vi "MENG4730 Flow Control By Valve Experiment.vi"() -> ()   [LabVIEW 2021]
uses:
  <vilib>/addons/control/pid/pid.llb/PID (DBL).vi
  <vilib>/Modbus/slave/Modbus Slave.lvclass
  <vilib>/addons/control/pid/NI_PID_pid.lvlib
panel:
  in  "FV1":bool
  out "x+1":dbl
  out "FV2":sgl
  out "F1 Values Array":dbl[](array[numeric])
  out "output":sgl
  in  "Flow Setpoint":dbl format="%.2f"
  out "Waveform Graph":sgl[](graph)
  in  "PID gains":T1={"proportional gain (Kc)"=1.0, "integral time (Ti, min)"=0.01, "derivative time (Td, min)"=0.0} {"derivative time (Td, min)" format="%.3f"; "integral time (Ti, min)" format="%.3f"; "proportional gain (Kc)" format="%.3f"}
  out "F1":sgl
  out "F1":sgl(knob) scale=0.0..100.0
  in  "stop":bool
  in  "M1":sgl(slide) scale=0.0..100.0
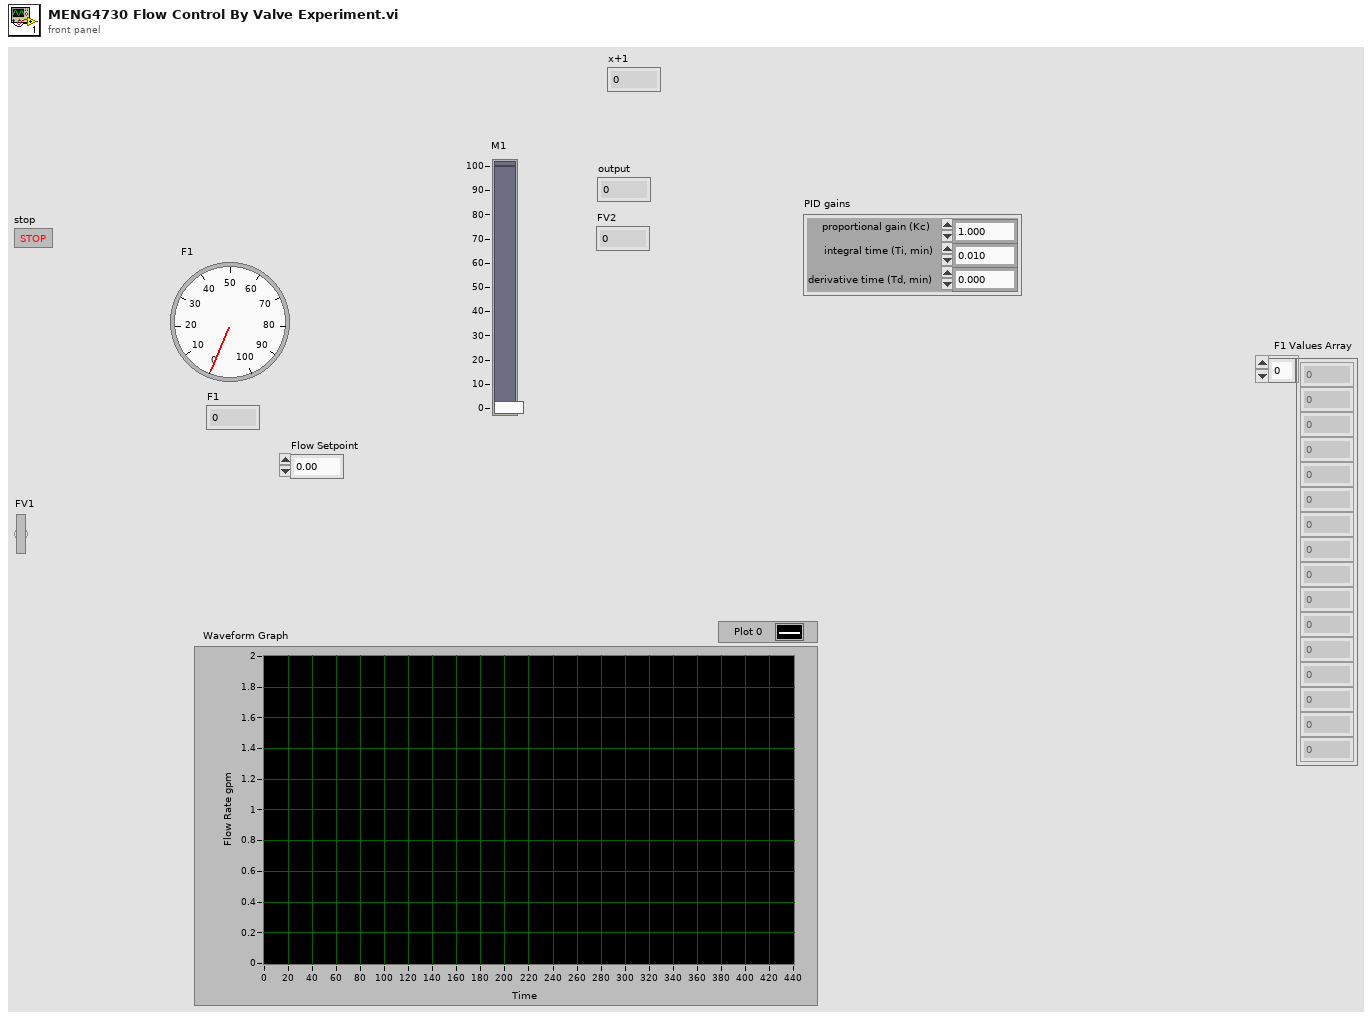
[diagram p1: front panel]
types:
  T1 = cluster{"proportional gain (Kc)":dbl, "integral time (Ti, min)":dbl, "derivative time (Td, min)":dbl}
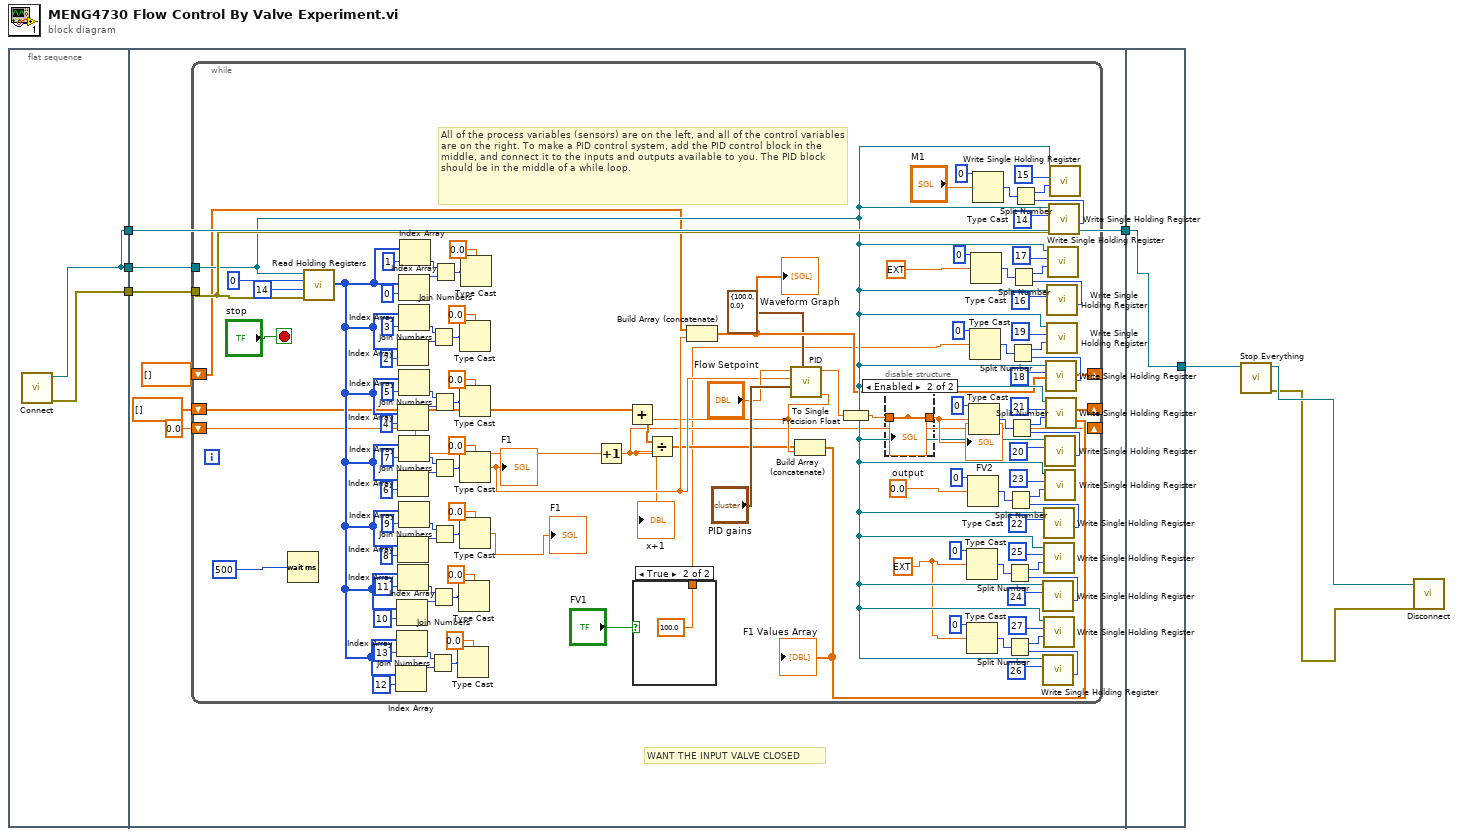
[diagram p0: block diagram]
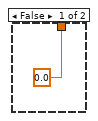
[diagram p2: hidden frame]
diagram:
  n1 = flat-sequence {
    tunnel: [w9] -> w7
    tunnel: [w8] -> w6
    tunnel: [w9] -> w5
    tunnel: w7 -> [w15]
    tunnel: w6 -> [w14]
    tunnel: [w13] -> w4
    tunnel: w5 -> [w13]
    tunnel: w4 -> [w133]
    tunnel: [w133] -> w3
    frame #0 {
      n2 = call "Connect.vi"() -> ("TCP slave instance"=w9:refnum<class "Modbus Slave.lvclass">, "error out"=w8:errorcluster)  [unwired: 8 in]
    }
    frame #1 {
      # "WANT THE INPUT VALVE CLOSED"
      n3 = while {
        tunnel: w15 -> [w37]
        tunnel: w14 -> [w125]
        shift-right: [w33] -> _
        shift-left: sgl[] [] -> [w34]
        shift-right: [w30] -> _
        shift-left: dbl[] [] -> [w22]
        shift-right: [w20] -> _
        shift-left: 0.0 -> [w21]
        stop <- "stop" stop-if-true
        w19 = ext 0.0 ("x")
        # "All of the process variables (sensors) are on the left, and all of the control variables are on the right. To make a PID control system, add the PID control block in the middle, and connect it to the inputs and outputs available to you. The PID block should be in the middle of a while loop."
        n4 = Wait (ms)(milliseconds to wait=u32 500) -> ()  [unwired: 1 out]
        n5 = call-dynamic "Read Holding Registers.vi"("error in (no error)"=w125, "number of holding registers"=u16 14, "starting address"=u16 0, "Modbus slave in"=w37) -> ("register values"=w76:u16[])  [unwired: 5 in, 2 out]
        n6 = Index Array(array=w76, index=12) -> (element=w78:u16)
        n7 = Index Array(array=w76, index=10) -> (element=w84:u16)
        n8 = Index Array(array=w76, index=13) -> (element=w77:u16)
        n9 = Index Array(array=w76, index=2) -> (element=w108:u16)
        n10 = Index Array(array=w76, index=4) -> (element=w102:u16)
        n11 = Index Array(array=w76, index=6) -> (element=w96:u16)
        n12 = Index Array(array=w76, index=8) -> (element=w90:u16)
        n13 = Index Array(array=w76, index=11) -> (element=w83:u16)
        n14 = Index Array(array=w76, index=0) -> (element=w114:u16)
        n15 = Index Array(array=w76, index=3) -> (element=w107:u16)
        n16 = Index Array(array=w76, index=5) -> (element=w101:u16)
        n17 = Index Array(array=w76, index=7) -> (element=w95:u16)
        n18 = Index Array(array=w76, index=9) -> (element=w89:u16)
        n19 = Index Array(array=w76, index=1) -> (element=w113:u16)
        n20 = Join Numbers(hi=w77, lo=w78) -> ((hi.lo)=w79:u32)
        n21 = Join Numbers(hi=w107, lo=w108) -> ((hi.lo)=w109:u32)
        n22 = Join Numbers(hi=w83, lo=w84) -> ((hi.lo)=w85:u32)
        n23 = Join Numbers(hi=w101, lo=w102) -> ((hi.lo)=w103:u32)
        n24 = Join Numbers(hi=w95, lo=w96) -> ((hi.lo)=w97:u32)
        n25 = Join Numbers(hi=w89, lo=w90) -> ((hi.lo)=w91:u32)
        n26 = Join Numbers(hi=w113, lo=w114) -> ((hi.lo)=w115:u32)
        n27 = Type Cast(type=sgl 0.0, x=w79) -> ()  [unwired: 1 out]
        n28 = Type Cast(type=sgl 0.0, x=w85) -> ()  [unwired: 1 out]
        n29 = Type Cast(type=sgl 0.0, x=w109) -> ()  [unwired: 1 out]
        n30 = Type Cast(type=sgl 0.0, x=w103) -> ()  [unwired: 1 out]
        n31 = Type Cast(type=sgl 0.0, x=w97) -> (*(type *) &x=w26:sgl)
        "F1" <- w26
        n32 = Type Cast(type=sgl 0.0, x=w91) -> (*(type *) &x=→"F1":sgl)
        n33 = Type Cast(type=sgl 0.0, x=w115) -> ()  [unwired: 1 out]
        n34 = Increment(x=w21) -> (x+1=w20:dbl)
        "x+1" <- w20
        n35 = case shown="True" "FV1" {
          tunnel: [sgl 0.0 ("FV1") sgl 100.0 ("FV1")] -> w16
          frame False {
          }
          frame True {
          }
        }
        n36 = Build Array (concatenate)(w34, w26) -> (w33:sgl[])
        "Waveform Graph" <- w33
        n37 = call-poly <vilib>:"PID.vi"("output range"=cluster{"output high":dbl, "output low":dbl} {"output high"=100.0, "output low"=0.0}, "PID gains"="PID gains", "process variable"=w26, "setpoint"="Flow Setpoint") -> ("dt out (s)"=w25:dbl, "output"=w29:dbl)  [unwired: 6 in]
        n38 = Add(x=w22, y=w25) -> (x+y=w24:dbl[])
        n39 = Divide(x=w24, y=w20) -> (x/y=w23:dbl[])
        n40 = Build Array (concatenate)(w23, w25) -> (w30:dbl[])
        "F1 Values Array" <- w30
        n41 = To Single Precision Float(number=w29) -> (single precision float=w28:sgl)
        n42 = disable-structure shown="Enabled" {
          disable-tunnel: [_ w132] -> w57
          disable-tunnel: w28 -> [_ w132]
          frame Disabled {
          }
          frame Enabled {
            "output" <- w132
          }
        }
        "FV2" <- w57
        n43 = Type Cast(type=u32 0, x=w19) -> (*(type *) &x=w45:u32)
        n44 = Type Cast(type=u32 0, x=w19) -> (*(type *) &x=w39:u32)
        n45 = Type Cast(type=u32 0, x=sgl 0.0 ("FV3")) -> (*(type *) &x=w52:u32)
        n46 = Type Cast(type=u32 0, x=w57) -> (*(type *) &x=w59:u32)
        n47 = Type Cast(type=u32 0, x=w16) -> (*(type *) &x=w65:u32)
        n48 = Type Cast(type=u32 0, x=ext 0.0) -> (*(type *) &x=w71:u32)
        n49 = Type Cast(type=u32 0, x="M1") -> (*(type *) &x=w121:u32)
        n50 = Split Number(x=w45) -> (hi(x)=w47:u16, lo(x)=w46:u16)
        n51 = Split Number(x=w39) -> (hi(x)=w41:u16, lo(x)=w40:u16)
        n52 = Split Number(x=w52) -> (hi(x)=w54:u16, lo(x)=w53:u16)
        n53 = Split Number(x=w59) -> (hi(x)=w61:u16, lo(x)=w60:u16)
        n54 = Split Number(x=w65) -> (hi(x)=w67:u16, lo(x)=w66:u16)
        n55 = Split Number(x=w71) -> (hi(x)=w73:u16, lo(x)=w72:u16)
        n56 = Split Number(x=w121) -> (hi(x)=w123:u16, lo(x)=w122:u16)
        n57 = call-dynamic "Write Single Holding Register.vi"("holding register value"=w46, "address"=u16 24, "Modbus slave in"=w37) -> ()  [unwired: 7 in, 2 out]
        n58 = call-dynamic "Write Single Holding Register.vi"("holding register value"=w40, "address"=u16 26, "Modbus slave in"=w37) -> ()  [unwired: 7 in, 2 out]
        n59 = call-dynamic "Write Single Holding Register.vi"("holding register value"=w53, "address"=u16 22, "Modbus slave in"=w37) -> ()  [unwired: 7 in, 2 out]
        n60 = call-dynamic "Write Single Holding Register.vi"("holding register value"=w47, "address"=u16 25, "Modbus slave in"=w37) -> ()  [unwired: 7 in, 2 out]
        n61 = call-dynamic "Write Single Holding Register.vi"("holding register value"=w41, "address"=u16 27, "Modbus slave in"=w37) -> ()  [unwired: 7 in, 2 out]
        n62 = call-dynamic "Write Single Holding Register.vi"("holding register value"=w60, "address"=u16 20, "Modbus slave in"=w37) -> ()  [unwired: 7 in, 2 out]
        n63 = call-dynamic "Write Single Holding Register.vi"("holding register value"=w54, "address"=u16 23, "Modbus slave in"=w37) -> ()  [unwired: 7 in, 2 out]
        n64 = call-dynamic "Write Single Holding Register.vi"("holding register value"=w66, "address"=u16 18, "Modbus slave in"=w37) -> ()  [unwired: 7 in, 2 out]
        n65 = call-dynamic "Write Single Holding Register.vi"("holding register value"=w61, "address"=u16 21, "Modbus slave in"=w37) -> ()  [unwired: 7 in, 2 out]
        n66 = call-dynamic "Write Single Holding Register.vi"("holding register value"=w72, "address"=u16 16, "Modbus slave in"=w37) -> ()  [unwired: 7 in, 2 out]
        n67 = call-dynamic "Write Single Holding Register.vi"("holding register value"=w67, "address"=u16 19, "Modbus slave in"=w37) -> ()  [unwired: 7 in, 2 out]
        n68 = call-dynamic "Write Single Holding Register.vi"("holding register value"=w73, "address"=u16 17, "Modbus slave in"=w37) -> ()  [unwired: 7 in, 2 out]
        n69 = call-dynamic "Write Single Holding Register.vi"("error in (no error)"=w125, "holding register value"=w122, "address"=u16 14, "Modbus slave in"=w37) -> ()  [unwired: 6 in, 2 out]
        n70 = call-dynamic "Write Single Holding Register.vi"("holding register value"=w123, "address"=u16 15, "Modbus slave in"=w37) -> ()  [unwired: 7 in, 2 out]
      }
    }
    frame #2 {
    }
  }
  n71 = call "Stop Everything.vi"("TCP slave instance"=w3) -> ("error out"=w1:errorcluster, "TCP slave instance"=w2:refnum<class "Modbus Slave.lvclass">)  [unwired: 9 in]
  n72 = call "Disconnect.vi"("error in (no error)"=w1, "TCP slave instance"=w2) -> ()  [unwired: 10 in]
